vi "EndOfLine_CRLF.vi"() -> (0 "String":string)   [LabVIEW 2012]
doc: "Begins a new line"
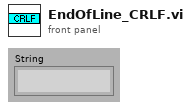
[diagram p1: front panel]
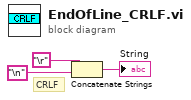
[diagram p0: block diagram]
diagram:
  # "CRLF"
  n1 = Concatenate Strings("\r", "\n") -> (→"String":string)
